vi "Generate Pretty Icon Text Layer.vi"(0 "Icon in":refnum<class "Icon.lvclass">, 5 "VI Name":string, 7 "Library Path":path, 9 "Number of Rows in Icon":i32, 11 "error in (no error)":errorcluster) -> (4 "Icon out":refnum<class "Icon.lvclass">, 15 "error out":errorcluster)   [LabVIEW 2020, in "Text-Based VI Icon.lvlib"]
doc: "Generating the LV Icon Text Layer requires the Text cluster.\nIn addition to the Text, it is possible to specify the visual appearance of the Text as well as a default Template Layer glyph.\n\nThe default value for the visual appearance is:\nFont: Small Fonts\nAlignment: Center\nSize: 8\nCenter text vertically: TRUE\nCapitalize text: TRUE\nColor of all four lines: Black\n\nThe default value of the Template layer is:\nSize: 32 x 32\nBorder Color: Black\nBackground Color: White"
uses:
  <vilib>/LabVIEW Icon API/Set Text Icon/Text-Based VI Icon.lvlib
  <vilib>/LabVIEW Icon API/lv_icon/Classes/Icon/Icon.lvclass
  <vilib>/LabVIEW Icon API/API_Test Settings.ctl
  <vilib>/LabVIEW Icon API/lv_icon/Controls/Alignment.ctl
  <vilib>/LabVIEW Icon API/API_Text Colors.ctl
  <vilib>/LabVIEW Icon API/lv_icon/Controls/Graphic.ctl
  <vilib>/LabVIEW Icon API/lv_icon/Classes/Icon Framework/Icon Framework.lvclass
  <vilib>/LabVIEW Icon API/LabVIEW Icon API.lvlib
panel:
  in  "LayerName":string="Icon Text"
  # "`"
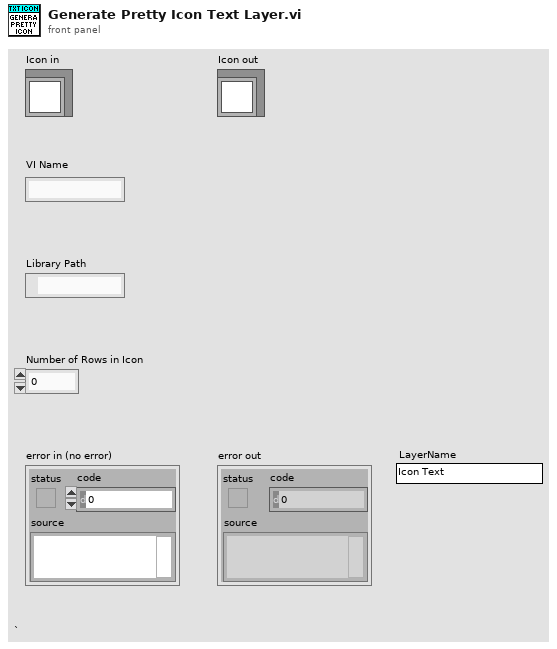
[diagram p1: front panel]
types:
  T1 = typedef "Graphic.ctl" = cluster{"Rectangle":cluster{"left":i16, "top":i16, "right":i16, "bottom":i16}, "Path":path, "Image":picture, "Filter":string, "FileName":string}
  T2 = typedef "LabVIEW Icon API.lvlib/API_Test Settings.ctl" = cluster{"Font":string, "Alignment":T3, "Size":u8, "Center text":bool, "Capitalize text":bool, "Text color":T4}
  T3 = typedef "Alignment.ctl" = u16
  T4 = typedef "LabVIEW Icon API.lvlib/API_Text Colors.ctl" = cluster{"Line 1 color":u32, "Line 2 color":u32, "Line 3 color":u32, "Line 4 color":u32}
  T5 = typedef "LabVIEW Icon API.lvlib/API_Text.ctl" = cluster{"Line 1 text":string, "Line 2 text":string, "Line 3 text":string, "Line 4 text":string}
  T6 = typedef "BodyText.ctl" = cluster{"Line 1 text":string, "Line 2 text":string, "Line 3 text":string, "Line 4 text":string, "Line 1 color":u32, "Line 2 color":u32, "Line 3 color":u32, "Line 4 color":u32, "Body Text Spec":cluster{"Font":T7, "Alignment":T3, "Size":u8}, "Center text vertically":bool, "Capitalize Text":bool}
  T7 = typedef "Font.ctl" = string
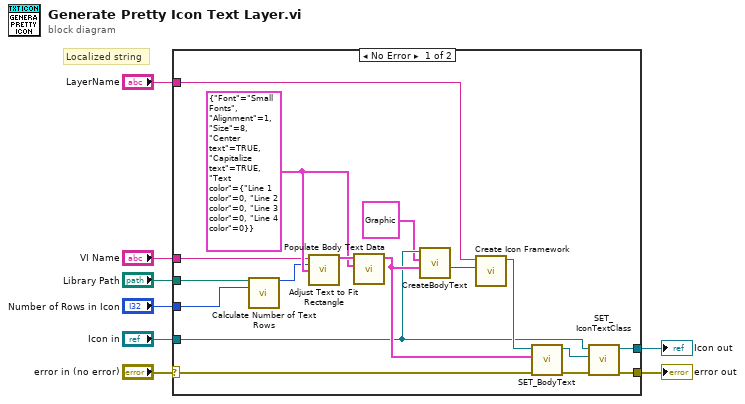
[diagram p0: block diagram]
diagram:
  # "Localized string"
  n1 = case shown="No Error" "error in (no error)" {
    selector: "error in (no error)" -> [w12 w27]
    tunnel: [w25 w27] -> w7
    tunnel: [w24 w26] -> w5
    tunnel: "Icon in" -> [w19 w26]
    tunnel: "VI Name" -> [w15 _]
    tunnel: "LayerName" -> [w13 _]
    tunnel: "Library Path" -> [w11 _]
    tunnel: "Number of Rows in Icon" -> [w10 _]
    frame No Error {
      w17 = T2 {"Font"="Small Fonts", "Alignment"=1, "Size"=8, "Center text"=TRUE, "Capitalize text"=TRUE, "Text color"={"Line 1 color"=0, "Line 2 color"=0, "Line 3 color"=0, "Line 4 color"=0}} ("Text settings")
      n2 = call <vilib>:"Calculate Number of Text Rows.vi"("Library Path"=w11, "Number of Pixel Rows in Icon"=w10) -> ("Number of Text Rows"=w9:i32)  [unwired: 13 in]
      n3 = call <vilib>:"Adjust Text to Fit Rectangle.vi"("VI Name"=w15, "Number of Rows"=w9, "Text settings"=w17) -> ("Text out"=w18:T5)  [unwired: 12 in]
      n4 = call <vilib>:"Populate Body Text Data.vi"("Text settings"=w17, "Text"=w18) -> ("Body Text"=w21:T6)  [unwired: 9 in]
      n5 = call <vilib>:"CreateBodyText.vi"("Body Text"=w21, "Path and Icon Template"=T1 {"Rectangle"={"left"=0, "top"=0, "right"=0, "bottom"=0}, "Path"=path "", "Image"=bytes[0], "Filter"="", "FileName"=""}, "Icon.lvclass in"=w19) -> ("Body Text"=w23:picture)  [unwired: 8 in]
      n6 = call <vilib>:"Create Icon Framework.vi"("Template Glyph"=w23, "Layer name"=w13) -> ("Icon Framework out"=w22:refnum<class "Icon Framework.lvclass">)  [unwired: 9 in]
      n7 = call-dynamic "SET_BodyText.vi"("error in (no error)"=w12, "Body Text"=w21, "Icon Framework.lvclass in"=w22) -> ("error out"=w14:errorcluster, "Icon Framework.lvclass out"=w20:refnum<class "Icon Framework.lvclass">)  [unwired: 7 in]
      n8 = call-dynamic "SET_IconTextClass.vi"("error in (no error)"=w14, "Icon Framework.lvclass"=w20, "Icon.lvclass in"=w19) -> ("error out"=w25:errorcluster, "Icon.lvclass out"=w24:refnum<class "Icon.lvclass">)  [unwired: 7 in]
    }
    frame Error {
    }
  }
  "error out" <- w7
  "Icon out" <- w5
